vi "Get AI Settings from AI TaskName in Dict.vi"(8 "error in (no error)":errorcluster, 10 "AI TaskName":string, 11 "DAQ":refnum<class "DAQ.lvclass">) -> (0 "error out":errorcluster, 2 "AI Settings":T1, 3 "DAQ":refnum<class "DAQ.lvclass">)   [LabVIEW 2017, in "DAQ.lvclass"]
doc: "Developed by Kevin Thompson\nkevin@thompsonengineering.net\n\nCopyright 2018-2020\nThompson Engineering, LLC"
uses:
  DAQ.lvclass
  DataTypes/TD AI Instrument Settings--cluster.ctl
  DataTypes/TD AI InstSettings--cluster.ctl
  Process/ProcessSupport/TD SimAI Ranges--cluster.ctl
  DAQ.lvclass/DAQ.ctl
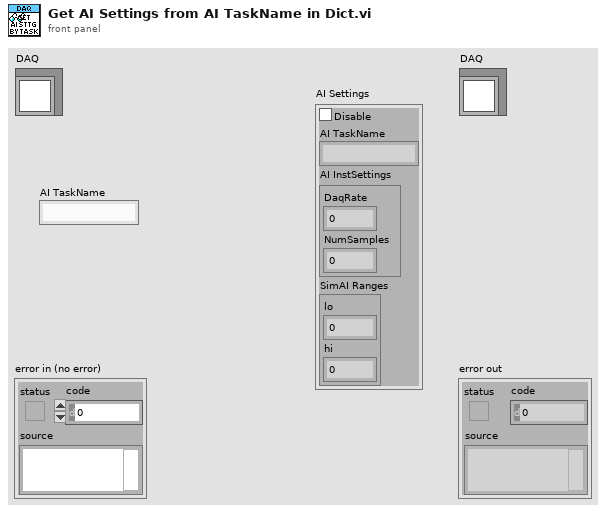
[diagram p1: front panel]
types:
  T1 = typedef "DAQ.lvclass/TD AI Instrument Settings--cluster.ctl" = cluster{"Disable":bool, "AI TaskName":string, "AI InstSettings":T2, "SimAI Ranges":T3}
  T2 = typedef "DAQ.lvclass/TD AI InstSettings--cluster.ctl" = cluster{"DaqRate":dbl, "NumSamples":i32}
  T3 = typedef "DAQ.lvclass/TD SimAI Ranges--cluster.ctl" = cluster{"lo":dbl, "hi":dbl}
  T4 = typedef "TD Dynamic CVT DVR--ref.ctl" = refnum<data-value>
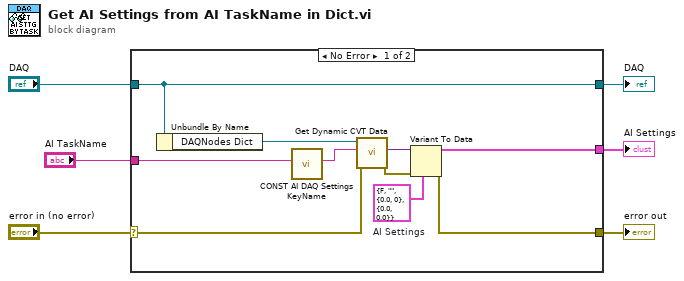
[diagram p0: block diagram]
diagram:
  n1 = case shown="No Error" "error in (no error)" {
    selector: "error in (no error)" -> [w14 w17]
    tunnel: [w13 w17] -> w5
    tunnel: [w16 w18] -> w3
    tunnel: "DAQ" -> [w16 w18]
    tunnel: "AI TaskName" -> [w10 _]
    tunnel: [w7 _] -> w1
    frame No Error {
      w8 = T1 {"Disable"=FALSE, "AI TaskName"="", "AI InstSettings"={"DaqRate"=0.0, "NumSamples"=0}, "SimAI Ranges"={"lo"=0.0, "hi"=0.0}}  # AI Settings
      n2 = Unbundle By Name(w16) -> ("DAQNodes Dict"=w15:T4)
      n3 = call "CONST AI DAQ Settings KeyName.vi"("AI TaskName"=w10) -> ("AI DAQ Settings (KeyName)"=w9:string)  [unwired: 10 in]
      n4 = call <vilib>:"Get Dynamic CVT Data.vi"("error in (no error)"=w14, "DataName"=w9, "dCVT DVR"=w15) -> ("error out"=w12:errorcluster, "value"=w11:variant)  [unwired: 5 in, 2 out]
      n5 = Variant To Data(error in=w12, type=w8, Variant=w11) -> (data=w7:T1, error out=w13:errorcluster)
    }
    frame Error {
    }
  }
  "error out" <- w5
  "DAQ" <- w3
  "AI Settings" <- w1
